vi "Preprocessing.vi"() -> (0 "Potência Ativa C":dbl[](graph), 1 "Potência Ativa B":dbl[](graph), 2 "Corrente C":dynamicdata(graph), 3 "Potência instantänea A":dbl[](array[numeric]), 4 "Corrente B":dynamicdata(graph), 5 "Tensão  C":dynamicdata(graph), 6 "Tensão B":dynamicdata(graph), 7 "Timestamp":dbl[](array[numeric]), 8 "Tensão A":dynamicdata(graph), 9 "Corrente A":dynamicdata(graph))   [LabVIEW 2024]
uses:
  <vilib>/numeric/Random Number (Range) DBL.vi
panel:
  out "Fator de potência":dbl
  out "Potência Ativa A":dbl[](graph)
  out "Corrente A":dbl[](array[numeric])
  out "Tensão A":dbl[](array[numeric])
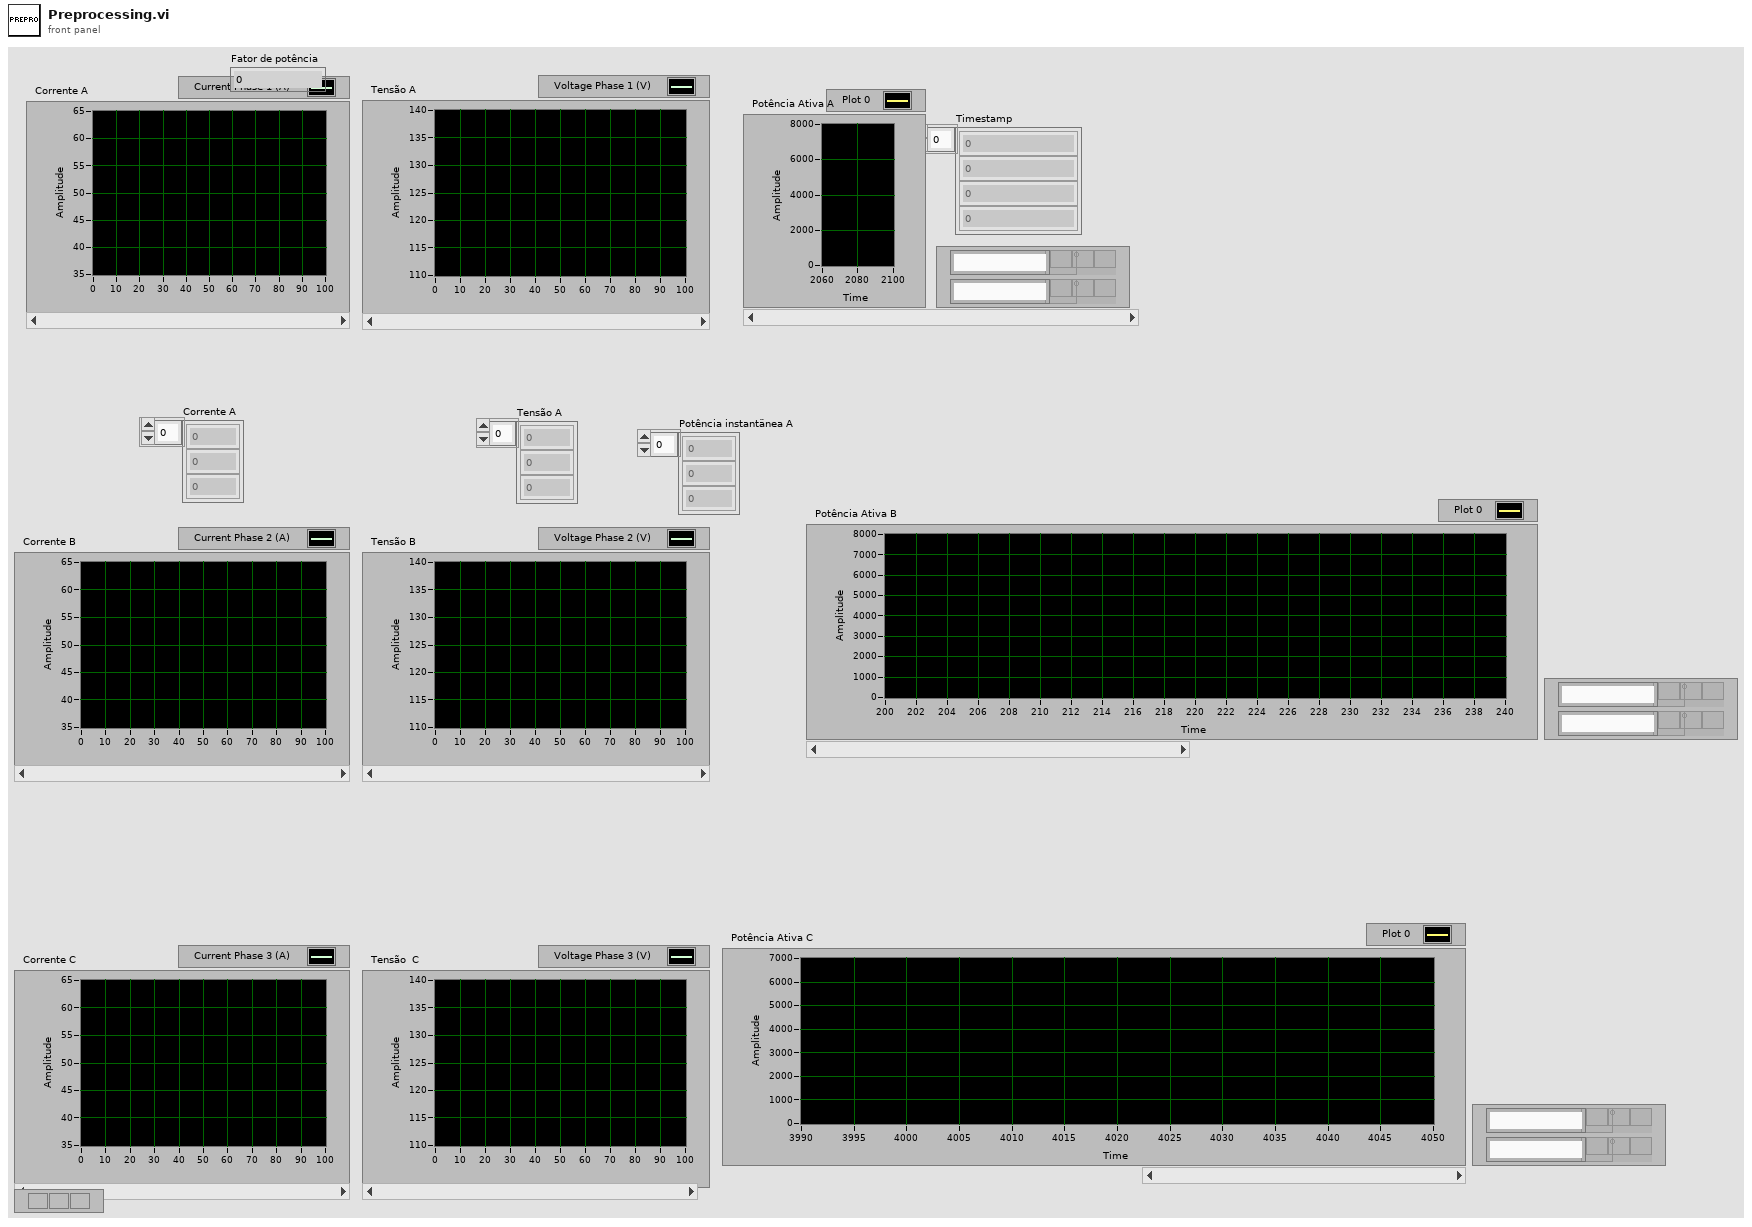
[diagram p1: front panel]
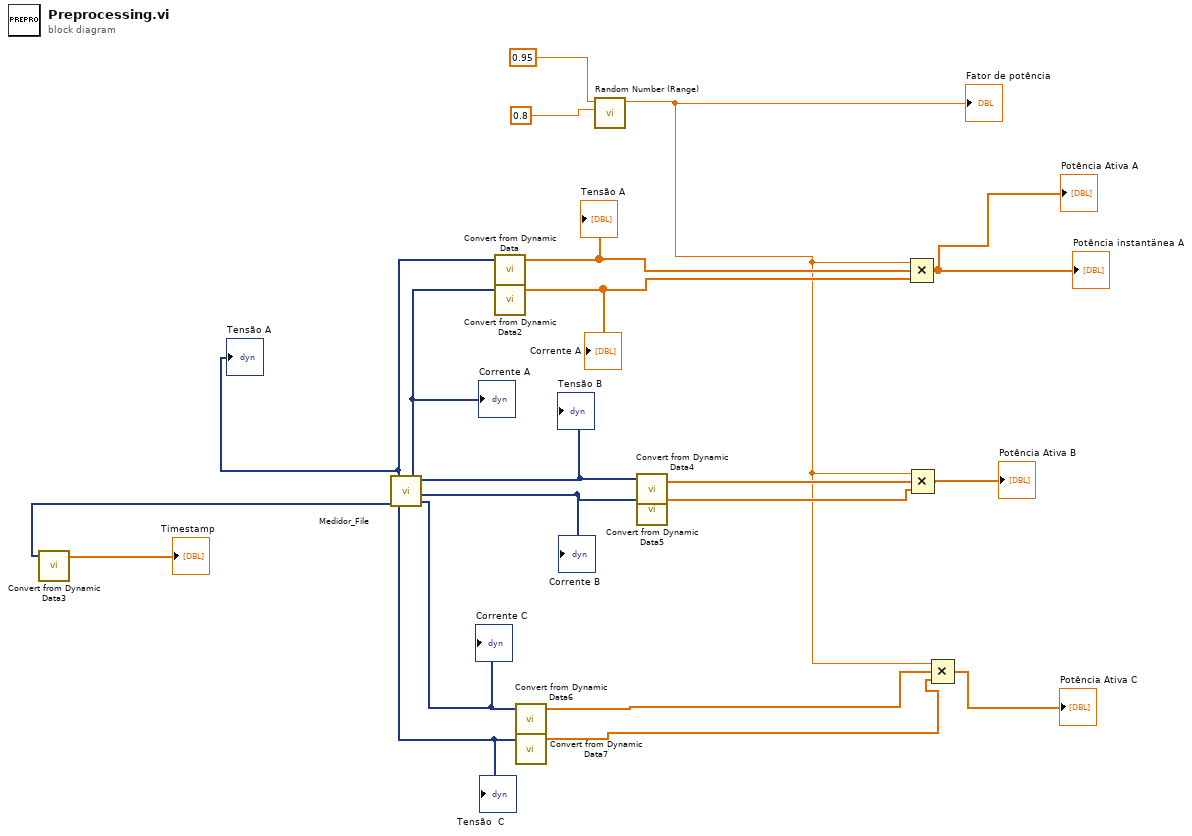
[diagram p0: block diagram]
diagram:
  n1 = call "Medidor_File.vi"() -> ("Corrente Fase C"=w9:dynamicdata, "Corrente Fase B"=w15:dynamicdata, "Corrente Fase A"=w7:dynamicdata, "TimeStamp"=w17:dynamicdata, "Tensão Fase C"=w10:dynamicdata, "Tensão Fase B"=w14:dynamicdata, "Tensão Fase A"=w20:dynamicdata)
  "Tensão A" <- w20
  "Corrente B" <- w15
  "Tensão B" <- w14
  "Corrente C" <- w9
  "Tensão  C" <- w10
  "Corrente A" <- w7
  n2 = call "Convert from Dynamic Data3"("Dynamic Data Type"=w17) -> ("Array"=→"Timestamp":dbl[])  [unwired: 3 in]
  n3 = call "Convert from Dynamic Data"("Dynamic Data Type"=w20) -> ("Array"=w19:dbl[])  [unwired: 3 in]
  "Tensão A" <- w19
  n4 = call "Convert from Dynamic Data2"("Dynamic Data Type"=w7) -> ("Array"=w18:dbl[])  [unwired: 3 in]
  "Corrente A" <- w18
  n5 = call "Convert from Dynamic Data6"("Dynamic Data Type"=w9) -> ("Array"=w4:dbl[])  [unwired: 3 in]
  n6 = call "Convert from Dynamic Data7"("Dynamic Data Type"=w10) -> ("Array"=w3:dbl[])  [unwired: 3 in]
  n7 = call-poly <vilib>:"Random Number (Range).vi"("lower bound (0)"=0.8 ("Limite superior FP"), "upper bound (100)"=0.95 ("Limite superior FP")) -> ("number"=w1:dbl)  [unwired: 9 in]
  "Fator de potência" <- w1
  n8 = call "Convert from Dynamic Data4"("Dynamic Data Type"=w14) -> ("Array"=w13:dbl[])  [unwired: 3 in]
  n9 = call "Convert from Dynamic Data5"("Dynamic Data Type"=w15) -> ("Array"=w12:dbl[])  [unwired: 3 in]
  n10 = Compound Arithmetic op=MULTIPLY(w1, w19, w18) -> (→"Potência instantänea A" →"Potência Ativa A":dbl[])
  n11 = Compound Arithmetic op=MULTIPLY(w1, w13, w12) -> (→"Potência Ativa B":dbl[])
  n12 = Compound Arithmetic op=MULTIPLY(w1, w4, w3) -> (→"Potência Ativa C":dbl[])
